vi "AM Send PS CMDs.vi"(6 "PS Index":enum16{"PS 1", "PS 2", "PS 3", "PS 4"}(ring), 9 "Current":dbl, 10 "Volt":dbl, 11 "Queue in":refnum<queue>) -> ()   [LabVIEW 2020, in "Motion.lvlib"]
uses:
  Motion.lvlib
  support/Message Queue/Message Queue.lvlib
  support/Message Queue/Enqueue Message (Single).vi
  support/Message Queue/Message Cluster.ctl
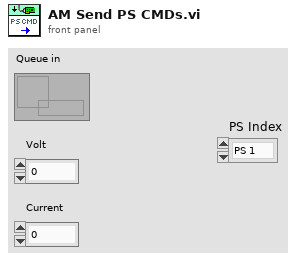
[diagram p1: front panel]
types:
  T1 = cluster{"Reset":bool, "PS Index":enum16{"PS 1", "PS 2", "PS 3", "PS 4"}}
  T2 = cluster{"Type":string, "Level":dbl, "PS Index":enum16{"PS 1", "PS 2", "PS 3", "PS 4"}}
  T3 = typedef "Message Queue.lvlib/Message Cluster.ctl" = cluster{"Message":string, "Message Data":variant}
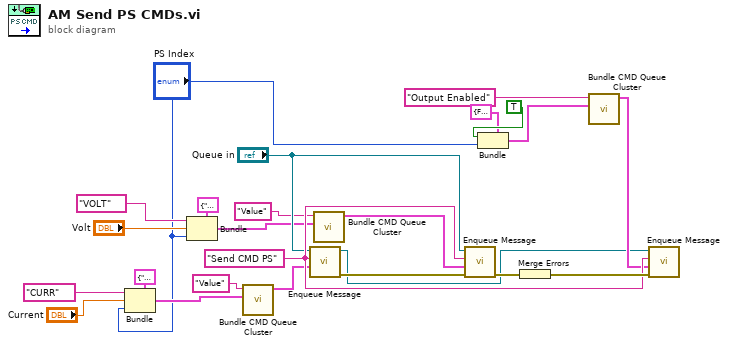
[diagram p0: block diagram]
diagram:
  w21 = "Send CMD PS" ("Message")
  n1 = Bundle(cluster=T2 {"Type"="", "Level"=0.0, "PS Index"=enum."PS 1"}, "Type"="CURR", "Level"="Current", "PS Index"="PS Index") -> (w6:T2)
  n2 = Bundle(cluster=T2 {"Type"="", "Level"=0.0, "PS Index"=enum."PS 1"}, "Type"="VOLT", "Level"="Volt", "PS Index"="PS Index") -> (w17:T2)
  n3 = call "Bundle CMD Queue Cluster.vi"("Message Data"=w6, "Message"="Value") -> ("Message Cluster"=w10:T3)  [unwired: 9 in]
  n4 = call-poly "Enqueue Message.vi"("Message Data"=w10, "Message"=w21, "Message Queue"="Queue in") -> ("error out"=w24:errorcluster, "dup Message Queue"=w11:refnum<queue>)  [unwired: 7 in]
  n5 = call "Bundle CMD Queue Cluster.vi"("Message Data"=w17, "Message"="Value") -> ("Message Cluster"=w19:T3)  [unwired: 9 in]
  n6 = call-poly "Enqueue Message.vi"("error in (no error)"=w24, "Message Data"=w19, "Message"=w21, "Message Queue"="Queue in") -> ("error out"=w22:errorcluster)  [unwired: 6 in, 1 out]
  n7 = Bundle(cluster=T1 {"Reset"=FALSE, "PS Index"=enum."PS 1"} ("output cluster"), "Reset"=TRUE, "PS Index"="PS Index") -> (w2:T1)
  n8 = Merge Errors(w22) -> (w23:errorcluster)
  n9 = call "Bundle CMD Queue Cluster.vi"("Message Data"=w2, "Message"="Output Enabled") -> ("Message Cluster"=w13:T3)  [unwired: 9 in]
  n10 = call-poly "Enqueue Message.vi"("error in (no error)"=w23, "Message Data"=w13, "Message"=w21, "Message Queue"=w11) -> ()  [unwired: 6 in, 2 out]
